vi "Get DI DAQ SMQ - array.vi"(8 "error in (no error)":errorcluster, 9 "AI TaskNames":string[](array[string]), 10 "AI Thread SMQs":variant) -> (0 "error out":errorcluster, 1 "AI DAQ SMQ []":refnum<queue>[](array[refnum]), 2 "AI Thread SMQs out":variant)   [LabVIEW 2017, in "DAQ.lvclass"]
doc: "Developed by Kevin Thompson\nkevin@thompsonengineering.net\n\nCopyright 2018-2020\nThompson Engineering, LLC"
uses:
  DAQ.lvclass
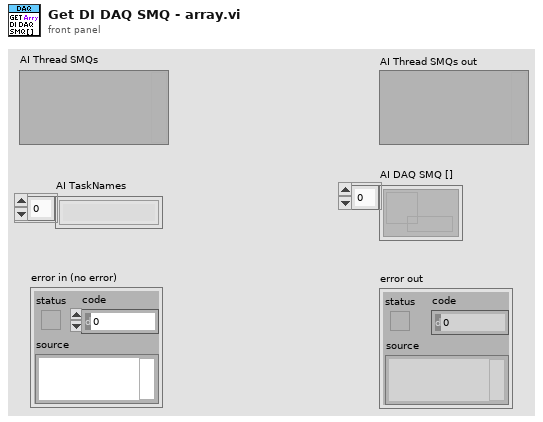
[diagram p1: front panel]
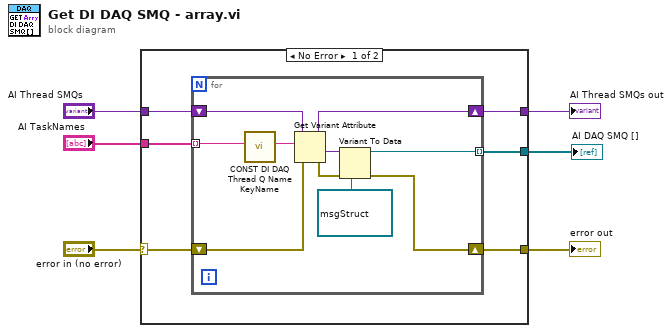
[diagram p0: block diagram]
diagram:
  n1 = case shown="No Error" "error in (no error)" {
    selector: "error in (no error)" -> [w11 w24]
    tunnel: [w10 w24] -> w5
    tunnel: "AI TaskNames" -> [w12 _]
    tunnel: "AI Thread SMQs" -> [w9 w23]
    tunnel: [w8 _] -> w2
    tunnel: [w7 w23] -> w3
    frame No Error {
      n2 = for {
        tunnel: w12 -> [w19] mode=indexing
        tunnel: [w14] -> w8 mode=indexing
        shift-right: [w16] -> w10
        shift-left: w11 -> [w17]
        shift-right: [w13] -> w7
        shift-left: w9 -> [w15]
        n3 = call "CONST DI DAQ Thread Q Name KeyName.vi"("DI TaskName"=w19) -> ("DI SMQ (KeyName)"=w20:string)  [unwired: 10 in]
        n4 = Get Variant Attribute(Variant=w15, name=w20, error in=w17) -> (duplicate Variant=w13:variant, value=w21:variant, error out=w18:errorcluster)  [unwired: 1 in, 1 out]
        n5 = Variant To Data(error in=w18, type=refnum<queue> refnum ("AI DAQ SMQ"), Variant=w21) -> (data=w14:refnum<queue>, error out=w16:errorcluster)
      }
    }
    frame Error {
    }
  }
  "error out" <- w5
  "AI Thread SMQs out" <- w3
  "AI DAQ SMQ []" <- w2
